vi "_CheckUserExist.vi"(8 "Error in":errorcluster caption="Error in (no error)", 11 "Username":string) -> (0 "Error out":errorcluster, 2 "exist？":bool, 3 "Username":string)   [LabVIEW 2017, in "Login-UI.lvlib"]
uses:
  Login-UI.lvlib
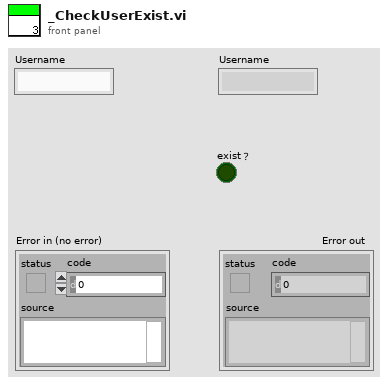
[diagram p1: front panel]
types:
  T1 = typedef "Login-UI.lvlib/User-Info.ctl" = cluster{"UserName":string, "Password":string, "Role":T2}
  T2 = typedef "Login-UI.lvlib/User-Role.ctl" = enum16{"INVALID", "Operator", "Engineer", "Admin"}
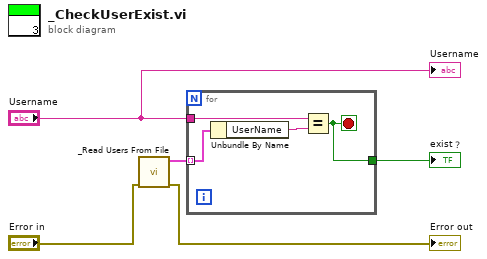
[diagram p0: block diagram]
diagram:
  n1 = call "_Read Users From File.vi"("Error in"="Error in") -> ("Error out"=→"Error out":errorcluster, "Array"=w5:T1[])  [unwired: 9 in]
  n2 = for {
    tunnel: w5 -> [w7] mode=indexing
    tunnel: "Username" -> [w9]
    tunnel: [w6] -> w1
    stop <- w6 stop-if-true
    n3 = Unbundle By Name(w7) -> ("UserName"=w8:string)
    n4 = Equal?(x=w9, y=w8) -> (x = y?=w6:bool)
  }
  "exist？" <- w1
  "Username" <- "Username"
